vi "Read_Write File.vi"(7 "Read/Write File":T2, 8 "error in":errorcluster, 9 "User Input":string="ATM accounts.txt", 10 "PIN_IN":string="ATM accounts.txt") -> (0 "error out":errorcluster, 1 "Output Value":string, 2 "Message type":string, 4 "PIN":string)   [LabVIEW 2019]
doc: "To take care of File for read and modification."
uses:
  controls/Read & Write File.ctl
  controls/Account Details.ctl
  <vilib>/Utility/file.llb/Write Delimited Spreadsheet (string).vi
  <vilib>/Utility/file.llb/Read Delimited Spreadsheet (string).vi
panel:
  out "Account":T1[](array[typedef])
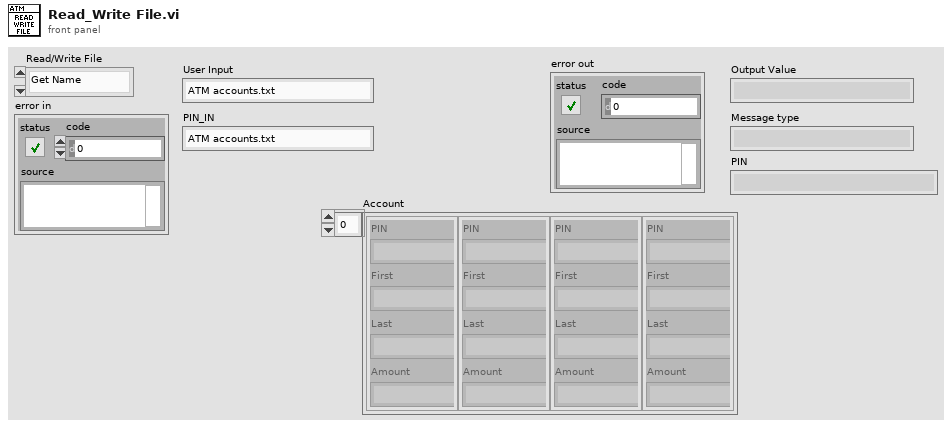
[diagram p1: front panel]
types:
  T1 = typedef "Account Details.ctl" = cluster{"PIN":string, "First":string, "Last":string, "Amount":string}
  T2 = typedef "Read & Write File.ctl" = enum16{"Get Name", "Update Balance", "Init", "Get Balance"}
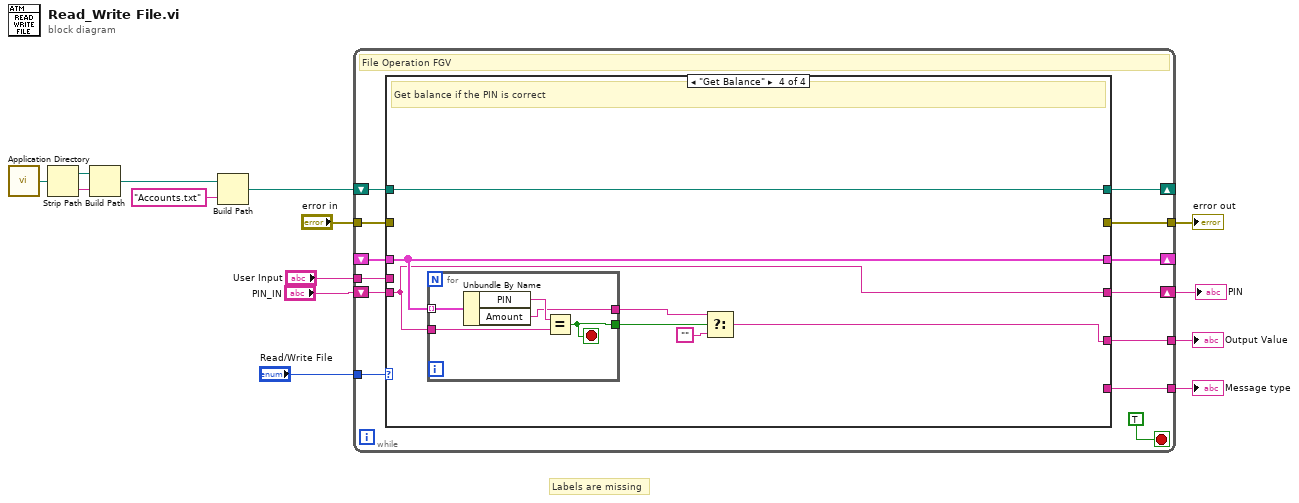
[diagram p0: block diagram]
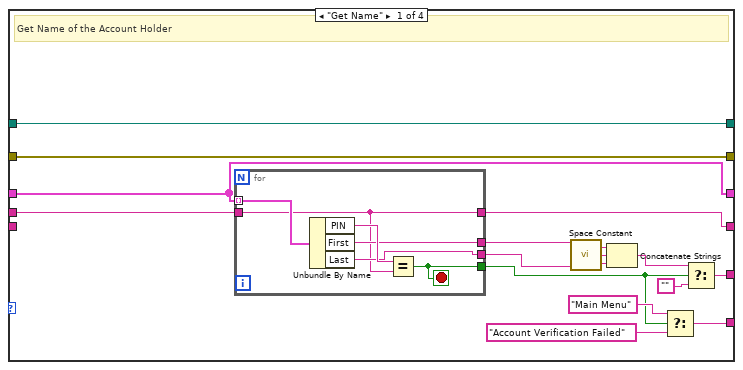
[diagram p2: hidden frame]
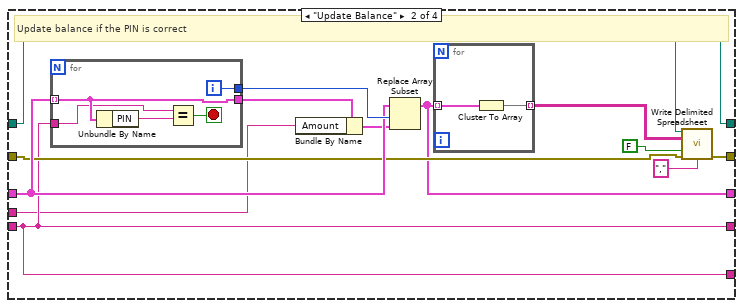
[diagram p3: hidden frame]
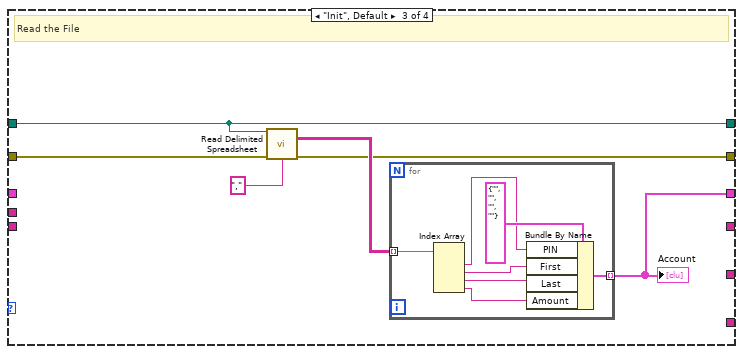
[diagram p4: hidden frame]
diagram:
  # "Labels are missing"
  n1 = call <vilib>:"Application Directory.vi"() -> ("Application Directory"=w11:path)
  n2 = Strip Path(path=w11) -> (stripped path=w10:path, name=w9:string)
  n3 = Build Path(base path=w10, name or relative path=w9) -> (appended path=w8:path)
  n4 = Build Path(base path=w8, name or relative path="Accounts.txt") -> (appended path=w6:path)
  n5 = while {
    tunnel: [w25] -> w13
    tunnel: "error in" -> [w24]
    tunnel: "Read/Write File" -> [w26]
    shift-right: [w22] -> _
    shift-left: _ -> [w21]
    tunnel: "User Input" -> [w18]
    tunnel: [w17] -> w2
    tunnel: [w20] -> w4
    shift-right: [w16] -> w1
    shift-left: "PIN_IN" -> [w19]
    shift-right: [w15] -> _
    shift-left: w6 -> [w23]
    stop <- TRUE stop-if-true
    # "File Operation FGV"
    n6 = case shown="\"Get Balance\"" w26 {
      tunnel: [w42 w61 w70 _] -> w25
      tunnel: w24 -> [w42 w57 w74 _]
      tunnel: w23 -> [w28 w49 w69 w82]
      tunnel: [w35 w52 w71 w88] -> w22
      tunnel: w21 -> [w35 w59 _ w88]
      tunnel: [w37 w54 _ w83] -> w20
      tunnel: w19 -> [_ w54 _ w87]
      tunnel: w18 -> [w29 w53 _ _]
      tunnel: [w31 _ _ _] -> w17
      tunnel: [w30 w54 _ w87] -> w16
      tunnel: [w28 w49 w69 w82] -> w15
      frame "Get Name" {
        # "Get Name of the Account Holder"
        n7 = for {
          tunnel: w35 -> [w48] mode=indexing
          tunnel: [w46] -> w41
          tunnel: w29 -> [w43]
          tunnel: [w45] -> w39
          tunnel: [w44] -> w32
          tunnel: [w43] -> w30
          stop <- w44 stop-if-true
          n8 = Unbundle By Name(w48) -> ("PIN"=w47:string, "First"=w46:string, "Last"=w45:string)
          n9 = Equal?(x=w47, y=w43) -> (x = y?=w44:bool)
        }
        n10 = call <vilib>:"Space Constant.vi"() -> ("String"=w40:string)
        n11 = Concatenate Strings(w41, w40, w39) -> (w38:string)
        n12 = Select(t="Main Menu" ("Message type"), s=w32, f="Account Verification Failed" ("t")) -> (s? t:f=w31:string)
        n13 = Select(t=w38, s=w32, f="") -> (s? t:f=w37:string)
      }
      frame "Update Balance" {
        # "Update balance if the PIN is correct"
        n14 = for {
          tunnel: w59 -> [w65] mode=indexing
          tunnel: [w66] -> w60
          tunnel: [w65] -> w51
          tunnel: w54 -> [w64]
          i -> [w66]
          stop <- w67 stop-if-true
          n15 = Unbundle By Name(w65) -> ("PIN"=w68:string)
          n16 = Equal?(x=w64, y=w68) -> (x = y?=w67:bool)
        }
        n17 = Bundle By Name(cluster=w51, "Amount"=w53) -> (w50:T1)
        n18 = Replace Array Subset(array=w59, new element=w50, index=w60) -> (w52:T1[])
        n19 = for {
          tunnel: w52 -> [w63] mode=indexing
          tunnel: [w62] -> w58 mode=indexing
          n20 = Cluster To Array(cluster=w63) -> (array=w62:string[])
        }
        n21 = call-poly <vilib>:"Write Delimited Spreadsheet.vi"("file path (dialog if empty)"=w49, "2D data"=w58, "append to file? (new file:F)"=FALSE, "error in (no error)"=w57, "delimiter (\\t)"="," ("delimiter (\\t)")) -> ("error out"=w61:errorcluster)  [unwired: 9 in, 1 out]
      }
      frame "Init", Default {
        # "Read the File"
        n22 = call-poly <vilib>:"Read Delimited Spreadsheet.vi"("file path (dialog if empty)"=w69, "error in (no error)"=w74, "delimiter (\\t)"="," ("delimiter (\\t)")) -> ("all rows"=w72:string[][], "error out"=w70:errorcluster)  [unwired: 7 in, 4 out]
        n23 = for {
          tunnel: w72 -> [w81] mode=indexing
          tunnel: [w75] -> w71 mode=indexing
          n24 = Index Array(array=w81) -> (element #1=w79:string, element #2=w78:string, element #3=w77:string, element #4=w76:string)  [unwired: 4 in]
          n25 = Bundle By Name(cluster=T1 {"PIN"="", "First"="", "Last"="", "Amount"=""} ("Account Details"), "PIN"=w79, "First"=w78, "Last"=w77, "Amount"=w76) -> (w75:T1)
        }
        "Account" <- w71
      }
      frame "Get Balance" {
        # "Get balance if the PIN is correct"
        n26 = for {
          tunnel: w88 -> [w93] mode=indexing
          tunnel: w87 -> [w92]
          tunnel: [w90] -> w84
          tunnel: [w89] -> w85
          stop <- w89 stop-if-true
          n27 = Unbundle By Name(w93) -> ("PIN"=w91:string, "Amount"=w90:string)
          n28 = Equal?(x=w91, y=w92) -> (x = y?=w89:bool)
        }
        n29 = Select(t=w84, s=w85, f="") -> (s? t:f=w83:string)
      }
    }
  }
  "error out" <- w13
  "Output Value" <- w4
  "Message type" <- w2
  "PIN" <- w1
